vi "phan_xy.vi"() -> ()   [LabVIEW 2019]
uses:
  <vilib>/Platform/TimedLoop/XDataNode/timing_clust.ctl
  <vilib>/Platform/TimedLoop/XDataNode/nitl_modes.ctl
  <vilib>/Platform/TimedLoop/XDataNode/wakeup.ctl
  <vilib>/platform/TimedLoop/XDataNode/XDataNode.xnode
  <vilib>/Platform/TimedLoop/XDataNode/XDNodeRunTimeDep.lvlib
  <vilib>/ptbypt/NI_PtbyPt.lvlib
panel:
  out "dem":dbl
  out "Vxdk":dbl
  out "Vydk":dbl
  in  "Kdv3":dbl
  in  "Kiv3":dbl=28.5
  in  "Kpv3":dbl=0.7
  in  "Kdv2":dbl
  in  "Kiv2":dbl=28.5
  in  "Kpv2":dbl=0.7
  out "Ts":dbl=10.0
  out "TOA DO 2":dbl[][](array[numeric])
  out "sailechxy":cluster{"e_x":dbl, "e_y":dbl}(graph)
  in  "Kdxy":dbl
  in  "Kixy":dbl
  in  "Kpxy":dbl=4.0
  in  "?":enum32{"DUONG 2", "DUONGTRON", "NHAP DIEM"}(tab)
  in  "xstart":dbl format="%#_13g"
  in  "xend":dbl=2.0
  in  "time2":dbl=10.0
  in  "R":dbl=0.8
  in  "phi_end":dbl=15.71
  in  "phi_start":dbl=3.14159 format="%#_13g"
  in  "time1":dbl=30.0
  in  "y2":dbl
  in  "x1":dbl
  in  "x2":dbl
  in  "time3":dbl=10.0
  in  "x3":dbl
  in  "y3":dbl
  in  "y1":dbl
  in  "x4":dbl
  in  "y4":dbl
  out "V_ph":dbl
  out "w_ph3":dbl
  out "w_ph2":dbl
  out "w_ph1":dbl
  in  "RESETMAP":bool=TRUE caption="Reset"
  out "duty3":dbl
  out "duty2":dbl
  out "duty1":dbl
  in  "RESET":bool
  out "Y_sp":dbl
  out "X_sp":dbl
  out "Y_ph":dbl
  out "X_ph":dbl
  out "Map":cluster{"Y":dbl[], "Y":dbl[]}[](graph)
  out "V3_sp":dbl
  out "V3_ph":dbl
  out "VAN TOC":T1(graph)
  in  "Kdv1":dbl
  in  "Kiv1":dbl=28.5
  in  "Kpv1":dbl=0.7
  out "V2_ph":dbl
  out "V1_ph":dbl
  out "V2_sp":dbl
  out "V1_sp":dbl
  in  "START":bool
  # "HE THONG"
  # "PID VI TRI"
  # "PID TOC DO"
  # "DUTY"
  # "VI TRI DIEU KHIEN\n(m)"
  # "VI TRI PHAN HOI\n(m)"
  # "TOC DO PHAN HOI (rad/s)"
  # "VAN TOC DIEU KHIEN\n(m/s)"
  # "VAN TOC PHAN HOI\n(m/s)"
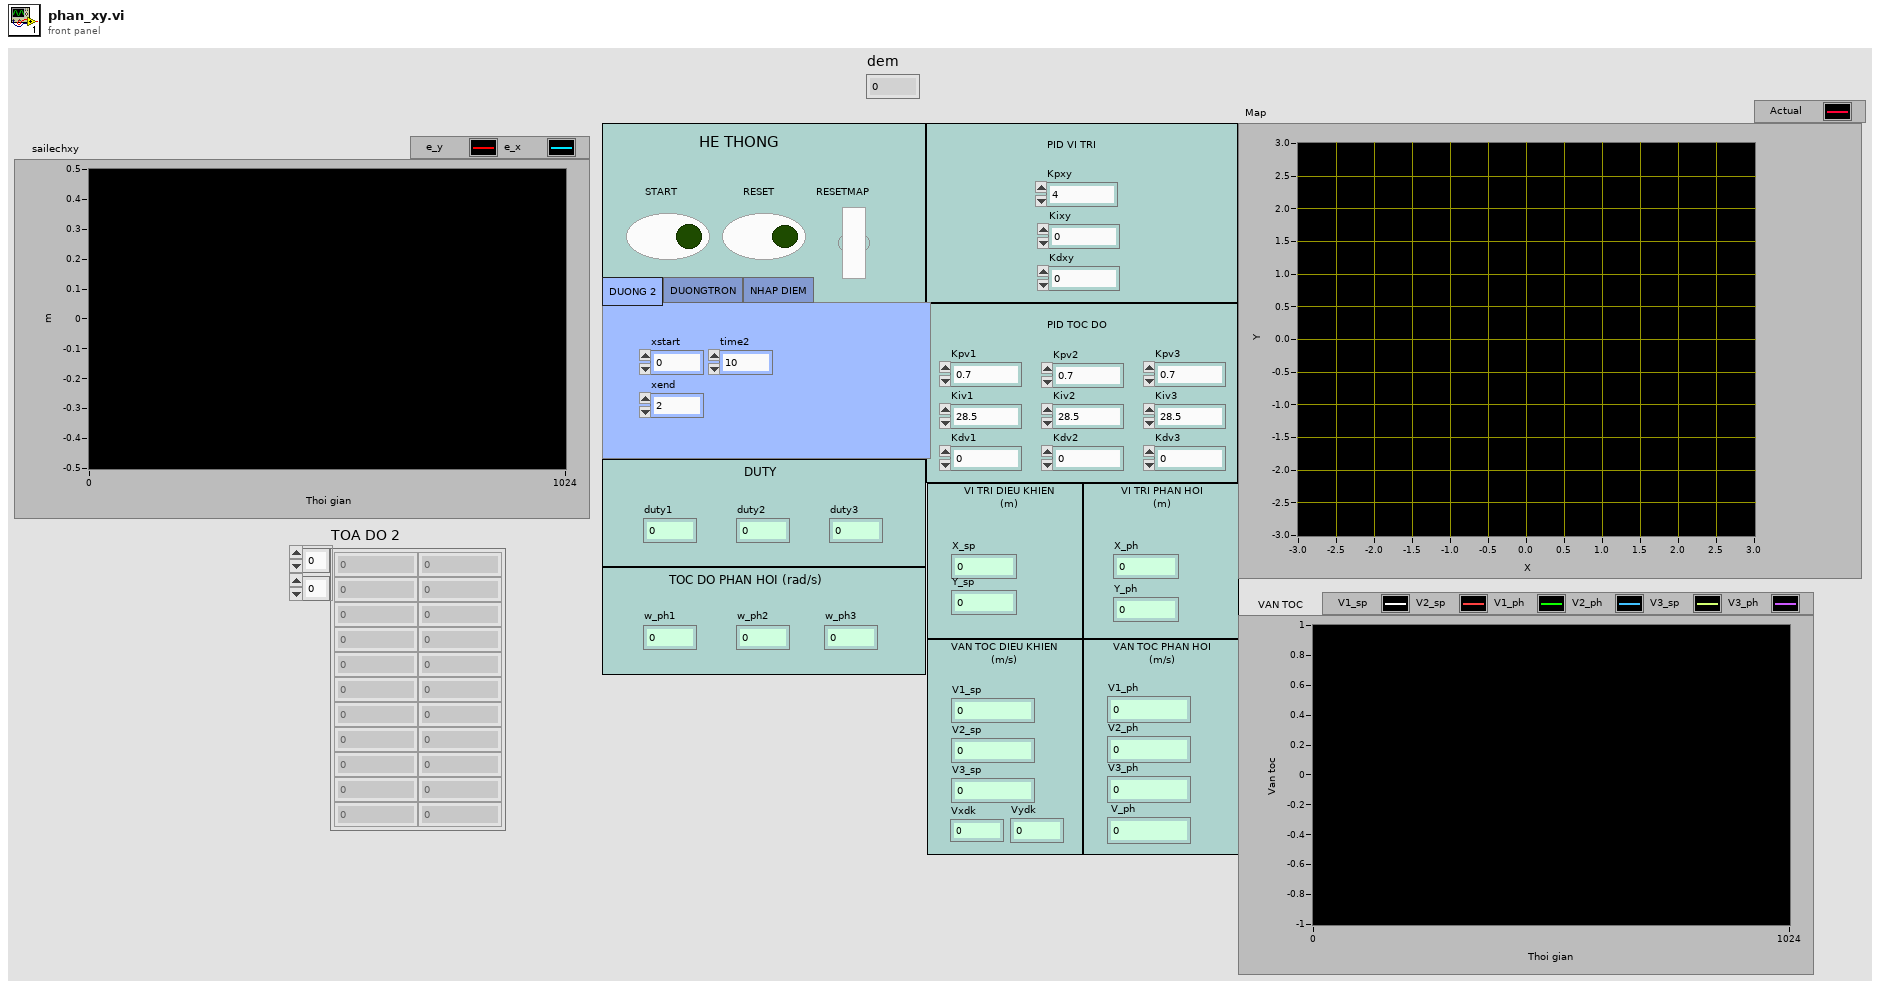
[diagram p1: front panel]
types:
  T1 = cluster{dbl, dbl, "V1_ph":dbl, "V2_ph":dbl, dbl, "V3_ph":dbl}
  T2 = typedef "XDNodeRunTimeDep.lvlib/timing_clust.ctl" = cluster{"Expected End [f-1]":u64, "Actual End [f-1]":u64, "Finished Late? [f-1]":bool, "Expected End [i-1]":u64, "Actual End [i-1]":u64, "Finished Late? [i-1]":bool, "Expected Start [i]":u64, "Actual Start [i]":u64, "Expected Start [f]":u64, "Actual Start [f]":u64, "Source Name":string, "Structure Name":string, "Period":i64, "Deadline":i64, "Offset":i64, "Start":i64, "Priority":i32, "Timeout":i32, "Mode":T3, "Wakeup Reason":T4, "Error":errorcluster, "Source Type":string, "Secondary Source Type":string, "Global End Time":u64, "Global Start Time":u64, "Frame Duration":u64, "Iteration Duration":u64, "Assigned CPU":i32, "I/O Scan Engine Mode":u32}
  T3 = typedef "XDNodeRunTimeDep.lvlib/nitl_modes.ctl" = enum32{"No Change", "Process missed periods, maintain original phase", "Discard missed periods, maintain original phase", "Process missed periods, ignore original phase", "Discard missed periods, ignore original phase"}
  T4 = typedef "XDNodeRunTimeDep.lvlib/wakeup.ctl" = enum32{"Normal", "Aborted", "Asynchronous wakeup", "Timing source error", "Timed loop error", "Timeout"}
  T5 = cluster{"V1_sp":dbl, "V_ph1":dbl, "V2_sp":dbl, "V_ph2":dbl, "V3_sp":dbl, "V_ph3":dbl}
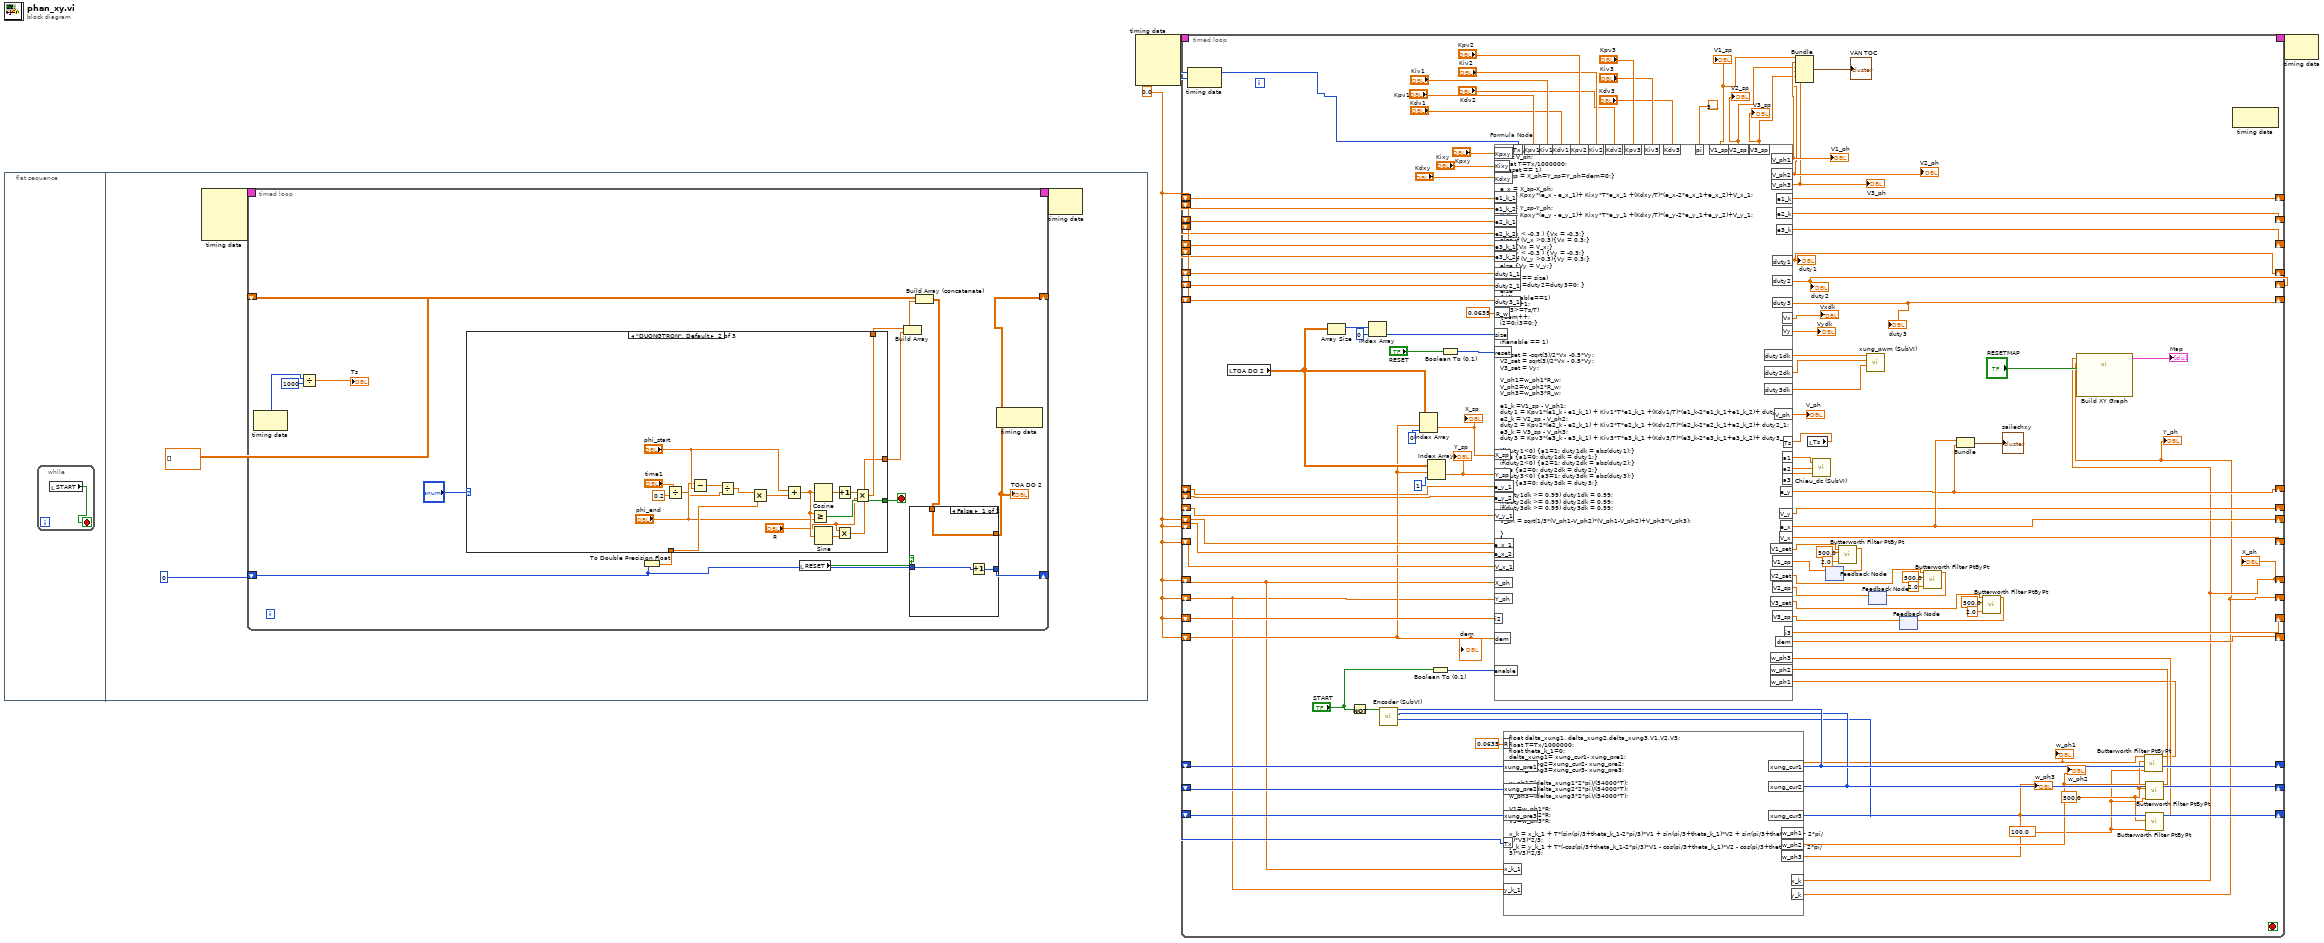
[diagram p0: block diagram]
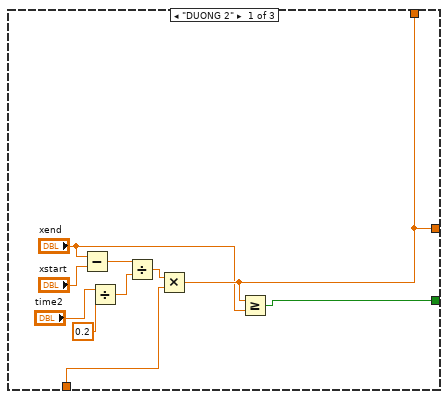
[diagram p2: hidden frame]
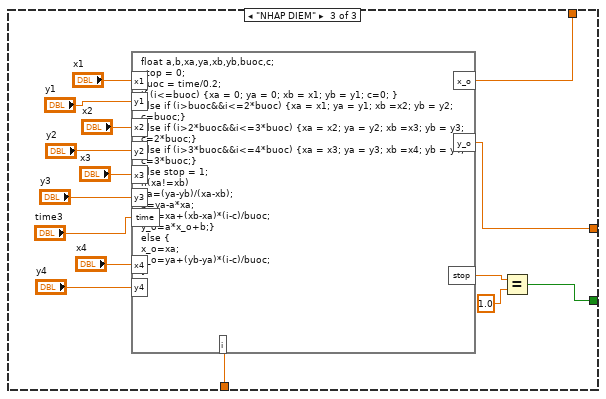
[diagram p3: hidden frame]
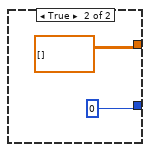
[diagram p4: hidden frame]
diagram:
  w1 = 0.0 ("e1")
  n1 = flat-sequence {
    frame #0 {
      n2 = while {
        stop <- w4 stop-if-true
        n3 = local read "START"() -> (w4:bool)
      }
    }
    frame #1 {
      n4 = node-c288() -> (w8:T2)  [unwired: 4 in]
      n5 = timed-loop {
        timing: w8 -> [_]
        timing-out: [_] -> w7
        shift-right: [w15] -> _
        shift-left: dbl[][] [] -> [w21]
        shift-right: [w19] -> _
        shift-left: 0 -> [w18]
        stop <- w12 stop-if-true
        n6 = node-c288() -> (w14:i64)  [unwired: 1 in]
        n7 = Divide(x=w14, y=i64 1000) -> (x/y=→"Ts":dbl)
        n8 = To Double Precision Float(number=w18) -> (double precision float=w23:dbl)
        n9 = case shown="\"DUONGTRON\", Default" "?" {
          tunnel: w23 -> [w30 w50 w65]
          tunnel: [w29 w44 w58] -> w17
          tunnel: [w29 w43 w53] -> w16
          tunnel: [w27 w42 w55] -> w12
          frame "DUONG 2" {
            n10 = Subtract(x="xend", y="xstart") -> (x-y=w32:dbl)
            n11 = Divide(x="time2", y=0.2) -> (x/y=w24:dbl)
            n12 = Divide(x=w32, y=w24) -> (x/y=w31:dbl)
            n13 = Multiply(x=w31, y=w30) -> (x*y=w29:dbl)
            n14 = Greater Or Equal?(x=w29, y="xend") -> (x >= y?=w27:bool)
          }
          frame "DUONGTRON", Default {
            n15 = Divide(x="time1", y=0.2) -> (x/y=w34:dbl)
            n16 = Subtract(x="phi_end", y="phi_start") -> (x-y=w38:dbl)
            n17 = Divide(x=w38, y=w34) -> (x/y=w37:dbl)
            n18 = Multiply(x=w37, y=w50) -> (x*y=w49:dbl)
            n19 = Add(x="phi_start", y=w49) -> (x+y=w48:dbl)
            n20 = Greater Or Equal?(x=w48, y="phi_end") -> (x >= y?=w42:bool)
            n21 = Cosine(x=w48) -> (cos(x)=w47:dbl)
            n22 = Sine(x=w48) -> (sin(x)=w45:dbl)
            n23 = Increment(x=w47) -> (x+1=w46:dbl)
            n24 = Multiply(x="R", y=w45) -> (x*y=w43:dbl)
            n25 = Multiply(x=w46, y="R") -> (x*y=w44:dbl)
          }
          frame "NHAP DIEM" {
            n26 = formula code="float a,b,xa,ya,xb,yb,buoc,c;\nstop = 0;\nbuoc = time/0.2;\nif (i<=buoc) {xa = 0; ya = 0; xb = x1; yb = y1; c=0; }\nelse if (i>buoc&&i<=2*buoc) {xa = x1; ya = y1; xb =x2; yb = y2; c=buoc;}\nelse if (i>2*buoc&&i<=3*buoc) {xa = x2; ya = y2; xb =x3; yb = y3; c=2*buoc;}\nelse if (i>3*buoc&&i<=4*buoc) {xa = x3; ya = y3; xb =x4; yb = y4; c=3*buoc;}\nelse stop = 1;\nif(xa!=xb)\n{a=(ya-yb)/(xa-xb);\nb=ya-a*xa;\nx_o=xa+(xb-xa)*(i-c)/buoc;\ny_o=a*x_o+b;}\nelse {\nx_o=xa;\ny_o=ya+(yb-ya)*(i-c)/buoc;\n}"("i"=w65, "x1"="x1", "y1"="y1", "x2"="x2", "y2"="y2", "x3"="x3", "y3"="y3", "time"="time3", "x4"="x4", "y4"="y4") -> ("x_o"=w58:dbl, "y_o"=w53:dbl, "stop"=w57:dbl)
            n27 = Equal?(x=w57, y=1.0) -> (x = y?=w55:bool)
          }
        }
        n28 = local read "RESET"() -> (w11:bool)
        n29 = Build Array(w17, w16) -> (w22:dbl[])
        n30 = Build Array (concatenate)(w21, w22) -> (w20:dbl[][])
        n31 = case shown="False" w11 {
          tunnel: w20 -> [w68 _]
          tunnel: [w68 dbl[][] []] -> w15
          tunnel: [w67 0] -> w19
          tunnel: w18 -> [w66 _]
          frame False {
            n32 = Increment(x=w66) -> (x+1=w67:i32)
          }
          frame True {
          }
        }
        "TOA DO 2" <- w15
        n33 = node-c288() -> ()  [unwired: 1 in, 1 out]
      }
      n34 = node-c288(w7) -> ()  [unwired: 1 out]
    }
  }
  n35 = node-c288() -> (w3:T2)  [unwired: 4 in]
  n36 = timed-loop {
    timing: w3 -> [_]
    timing-out: [_] -> w2
    shift-right: [w186] -> _
    shift-left: w1 -> [w184]
    shift-right: [w185] -> _
    shift-left: w1 -> [w140]
    shift-right: [w177] -> _
    shift-left: w1 -> [w176]
    shift-right: [w79] -> _
    shift-left: w1 -> [w77]
    shift-right: [w78] -> _
    shift-left: w1 -> [w76]
    shift-right: [w175] -> _
    shift-left: w1 -> [w108]
    shift-right: [w155] -> _
    shift-left: w1 -> [w156]
    shift-right: [w154] -> _
    shift-left: w1 -> [w151]
    shift-right: [w153] -> _
    shift-left: w1 -> [w150]
    shift-right: [w152] -> _
    shift-left: w1 -> [w149]
    shift-right: [w143] -> _
    shift-left: _ -> [w146]
    shift-right: [w142] -> _
    shift-left: _ -> [w145]
    shift-right: [w141] -> _
    shift-left: _ -> [w144]
    shift-right: [w91] -> _
    shift-left: w1 -> [w135]
    shift-right: [w133] -> _
    shift-left: w1 -> [w134]
    shift-left: w1 -> [w129]
    shift-left: w1 -> [w128]
    shift-left: w1 -> [w127]
    shift-left: w1 -> [w126]
    shift-right: [w82] -> _
    shift-left: _ -> [w87]
    shift-right: [w89] -> _
    shift-left: _ -> [w88]
    shift-left: _ -> [w86]
    stop <- _ stop-if-true
    w120 = 100.0 ("flw")
    w121 = 500.0 ("sampling freq: fs")
    n37 = node-c288() -> (w81:i64)  [unwired: 1 in]
    n38 = local read "TOA DO 2"() -> (w109:dbl[][])
    n39 = Array Size(array=w109) -> (size(s)=w171:i32[])
    n40 = Not(x="START") -> (.not. x?=w158:bool)
    n41 = Index Array(array=w171, index=0) -> (element=w169:i32)
    n42 = call "Encoder (SubVI).vi"("Boolean"=w158) -> ("Counter Value3"=w141:i32, "Counter Value 2"=w142:i32, "Counter Value"=w143:i32)  [unwired: 8 in]
    n43 = Index Array(array=w109, index (row)=w108, index (col)=0 ("disabled index (col)")) -> (element=w173:dbl)
    "X_sp" <- w173
    n44 = Index Array(array=w109, index (row)=w108, index (col)=1 ("disabled index (col)")) -> (element=w172:dbl)
    "Y_sp" <- w172
    n45 = Boolean To (0,1)(Boolean="START") -> (0, 1=w183:i16)
    n46 = Boolean To (0,1)(Boolean="RESET") -> (0, 1=w168:i16)
    n47 = formula code="float delta_xung1, delta_xung2,delta_xung3,V1,V2,V3;\nfloat T=Tx/1000000;\nfloat theta_k_1=0;\ndelta_xung1= xung_cur1- xung_pre1;\ndelta_xung2=xung_cur2- xung_pre2;\ndelta_xung3=xung_cur3- xung_pre3; \n\nw_ph1=(delta_xung1*2*pi)/(54000*T);\nw_ph2=(delta_xung2*2*pi)/(54000*T);\nw_ph3=(delta_xung3*2*pi)/(54000*T);\n\nV1=w_ph1*R;\nV2=w_ph2*R;\nV3=w_ph3*R;\n\nx_k = x_k_1 + T*(sin(pi/3+theta_k_1-2*pi/3)*V1 + sin(pi/3+theta_k_1)*V2 + sin(pi/3+theta_k_1 + 2*pi/3)*V3)*2/3;\ny_k = y_k_1 + T*(-cos(pi/3+theta_k_1-2*pi/3)*V1 - cos(pi/3+theta_k_1)*V2 - cos(pi/3+theta_k_1 + 2*pi/3)*V3)*2/3;"("xung_pre1"=w146, "xung_pre2"=w145, "xung_pre3"=w144, "xung_cur1"=w143, "xung_cur2"=w142, "xung_cur3"=w141, "Tx"=w81, "R"=0.0635 ("input variable"), "x_k_1"=w77, "y_k_1"=w76) -> ("w_ph1"=w111:dbl, "w_ph2"=w123:dbl, "w_ph3"=w122:dbl, "x_k"=w79:dbl, "y_k"=w78:dbl)
    "X_ph" <- w79
    "Y_ph" <- w78
    "w_ph1" <- w111
    "w_ph2" <- w123
    "w_ph3" <- w122
    n48 = local read "Ts"() -> (w83:dbl)
    n49 = feedback #1() -> (w99:dbl)  [unwired: 1 in]
    n50 = feedback #2() -> (w96:dbl)  [unwired: 1 in]
    n51 = feedback #3() -> (w93:dbl)  [unwired: 1 in]
    n52 = call "Build XY Graph"("Reset"="RESETMAP", "Y Input"=w78, "X Input"=w79) -> ("XY Graph"=→"Map":cluster{"X":dbl[], "Y":dbl[]}[])  [unwired: 7 in, 1 out]
    n53 = call <vilib>:"Butterworth Filter PtByPt.vi"("low cutoff freq: fl"=w120, "sampling freq: fs"=w121, "x"=w111) -> ("Filtered x"=w110:dbl)  [unwired: 6 in, 1 out]
    n54 = call <vilib>:"Butterworth Filter PtByPt.vi"("low cutoff freq: fl"=w120, "sampling freq: fs"=w121, "x"=w123) -> ("Filtered x"=w119:dbl)  [unwired: 6 in, 1 out]
    n55 = call <vilib>:"Butterworth Filter PtByPt.vi"("low cutoff freq: fl"=w120, "sampling freq: fs"=w121, "x"=w122) -> ("Filtered x"=w118:dbl)  [unwired: 6 in, 1 out]
    n56 = formula code="float V,Vtest, S_sp, S_ph, Vx, Vy;\nfloat V_ph;\n float T=Tx/1000000;\nif(reset == 1)\n{X_sp = X_ph=Y_sp=Y_ph=dem=0;}\n\ne_x = X_sp-X_ph; \nV_x = Kpxy*(e_x - e_x_1)+ Kixy*T*e_x_1 +(Kdxy/T)*(e_x-2*e_x_1+e_x_2)+V_x_1;\n\ne_y = Y_sp-Y_ph; \nV_y = Kpxy*(e_y - e_y_1)+ Kixy*T*e_y_1 +(Kdxy/T)*(e_y-2*e_y_1+e_y_2)+V_y_1;\n\n\nif (V_x < -0.3 ) {Vx = -0.3;} \nelse if (V_x >0.3){Vx = 0.3;}\nelse {Vx = V_x;}\nif (V_y < -0.3 ) {Vy = -0.3;} \nelse if (V_y >0.3){Vy = 0.3;}\nelse {Vy = V_y;}\n\nif(dem == size)\n{duty1=duty2=duty3=0; }\nelse\n{ if(enable==1)\n i3=i2+1;\nif (i3>=Ts/T)\n{dem++;\ni2=0;i3=0;}\n\n\nif(enable == 1)\n{\nV1_set = -sqrt(3)/2*Vx -0.5*Vy;\nV2_set = sqrt(3)/2*Vx - 0.5*Vy;\nV3_set = Vy; \n\nV_ph1=w_ph1*R_w;\nV_ph2=w_ph2*R_w;\nV_ph3=w_ph3*R_w;\n\ne1_k =V1_sp - V_ph1;\nduty1 = Kpv1*(e1_k - e1_k_1) + Kiv1*T*e1_k_1 +(Kdv1/T)*(e1_k-2*e1_k_1+e1_k_2)+ duty1_1;\ne2_k = V2_sp - V_ph2;\nduty2 = Kpv2*(e2_k - e2_k_1) + Kiv2*T*e2_k_1 +(Kdv2/T)*(e2_k-2*e2_k_1+e2_k_2)+ duty2_1;\ne3_k = V3_sp - V_ph3;\nduty3 = Kpv3*(e3_k - e3_k_1) + Kiv3*T*e3_k_1 +(Kdv3/T)*(e3_k-2*e3_k_1+e3_k_2)+ duty3_1;\n\nif(duty1<0) {a1=1; duty1dk = abs(duty1);}\nelse {a1=0; duty1dk = duty1;}\nif(duty2<0) {a2=1; duty2dk = abs(duty2);}\nelse {a2=0; duty2dk = duty2;}\nif(duty3<0) {a3=1; duty3dk = abs(duty3);}\nelse {a3=0; duty3dk = duty3;}\n\nif(duty1dk >= 0.99) duty1dk = 0.99;\nif(duty2dk >= 0.99) duty2dk = 0.99;\nif(duty3dk >= 0.99) duty3dk = 0.99;\n\nV_ph = sqrt(1/3*(V_ph1-V_ph2)*(V_ph1-V_ph2)+V_ph3*V_ph3);\n\n}\n}"("Kpv1"="Kpv1", "Kiv1"="Kiv1", "Kdv1"="Kdv1", "pi"=3.141592653589793, "e1_k_1"=w184, "e2_k_1"=w140, "enable"=w183, "Tx"=w81, "e3_k_1"=w176, "X_ph"=w77, "X_sp"=w173, "Y_sp"=w172, "Y_ph"=w76, "dem"=w108, "size"=w169, "reset"=w168, "i2"=w156, "duty1_1"=w151, "duty2_1"=w150, "duty3_1"=w149, "w_ph1"=w110, "w_ph2"=w119, "w_ph3"=w118, "e_x_1"=w135, "V_x_1"=w134, "Kpxy"="Kpxy", "Kixy"="Kixy", "Kdxy"="Kdxy", "e1_k_2"=w129, "e2_k_2"=w128, "e3_k_2"=w127, "e_x_2"=w126, "Ts"=w83, "Kpv2"="Kpv2", "Kiv2"="Kiv2", "Kdv2"="Kdv2", "Kpv3"="Kpv3", "Kiv3"="Kiv3", "Kdv3"="Kdv3", "V1_sp"=w99, "V2_sp"=w96, "V3_sp"=w93, "R_w"=0.0635 ("input variable"), "e_y_1"=w87, "e_y_2"=w86, "V_y_1"=w88) -> ("V1_sp"=w166:dbl, "V_ph1"=w165:dbl, "V_ph2"=w163:dbl, "e1_k"=w186:dbl, "e2_k"=w185:dbl, "V2_sp"=w164:dbl, "duty1"=w154:dbl, "duty2"=w153:dbl, "e3_k"=w177:dbl, "V_ph3"=w162:dbl, "V3_sp"=w161:dbl, "duty3"=w152:dbl, "a1"=w157:dbl, "a2"=w148:dbl, "a3"=w147:dbl, "dem"=w175:dbl, "i3"=w155:dbl, "duty1dk"=w139:dbl, "duty2dk"=w138:dbl, "duty3dk"=w137:dbl, "V_ph"=→"V_ph":dbl, "e_x"=w91:dbl, "V_x"=w133:dbl, "V1_set"=w101:dbl, "V2_set"=w98:dbl, "V3_set"=w95:dbl, "e_y"=w82:dbl, "V_y"=w89:dbl, "Vx"=→"Vxdk":dbl, "Vy"=→"Vydk":dbl)
    "V1_sp" <- w166
    "V2_sp" <- w164
    "V1_ph" <- w165
    "V2_ph" <- w163
    "V3_ph" <- w162
    "V3_sp" <- w161
    "duty1" <- w154
    "duty2" <- w153
    "duty3" <- w152
    n57 = Bundle("V1_sp"=w166, "V_ph1"=w165, "V2_sp"=w164, "V_ph2"=w163, "V3_sp"=w161, "V_ph3"=w162) -> (→"VAN TOC":T5)  [unwired: 1 in]
    n58 = call "Chieu_dc (SubVI).vi"("a3"=w147, "a2"=w148, "a1"=w157) -> ()
    n59 = call <vilib>:"Butterworth Filter PtByPt.vi"("low cutoff freq: fl"=2.0, "sampling freq: fs"=500.0, "x"=w101) -> ("Filtered x"=w100:dbl)  [unwired: 6 in, 1 out]
    n60 = feedback-in #1(w100) -> ()
    n61 = call "xung_pwm (SubVI).vi"("duty3 in"=w137, "duty2 in"=w138, "duty1 in"=w139) -> ()  [unwired: 6 in, 3 out]
    n62 = call <vilib>:"Butterworth Filter PtByPt.vi"("low cutoff freq: fl"=2.0, "sampling freq: fs"=500.0, "x"=w98) -> ("Filtered x"=w97:dbl)  [unwired: 6 in, 1 out]
    n63 = feedback-in #2(w97) -> ()
    n64 = Bundle("e_x"=w91, "e_y"=w82) -> (→"sailechxy":cluster{"e_x":dbl, "e_y":dbl})  [unwired: 1 in]
    n65 = call <vilib>:"Butterworth Filter PtByPt.vi"("low cutoff freq: fl"=2.0, "sampling freq: fs"=500.0, "x"=w95) -> ("Filtered x"=w94:dbl)  [unwired: 6 in, 1 out]
    n66 = feedback-in #3(w94) -> ()
    n67 = node-c288() -> ()  [unwired: 1 in, 1 out]
    "dem" <- w108
  }
  n68 = node-c288(w2) -> ()  [unwired: 1 out]
